vi "TEST_PumpController.vi"() -> ()   [LabVIEW 2024]
doc: "The purpose of this VI is for unit test of the Pump Controller"
uses:
  Control Definitions/Def PumpCtlRefs.ctl
  Control Definitions/Def PumpCtlOutputs.ctl
panel:
  in  "Pump Speed":enum16{"FAST", "SLOW", "CREEP", "STOP"}(ring)=enum."CREEP"
  in  "Bounds In":cluster{"Spec HI in":dbl, "Spec Lo in":dbl}={"Spec HI in"=7.5, "Spec Lo in"=7.4}
  out "outputs":T1={"PV"=2.1, "Done"=FALSE, "Over Fill"=FALSE, "Over Drain"=FALSE} {"PV" scale=0.0..10.0}
  in  "Level PV":dbl
  in  "Drain":bool
  in  "Fill":bool
  in  "Run Test":bool
  in  "Jog":bool
  in  "Pump CtlRef In":T2
  in  "Sim SwP":dbl=7.44 format="%_5g"
  in  "BinSearch":bool
  in  "Sim Pump":bool=TRUE
  in  "PV":dbl(slide)=2.1 scale=0.0..10.0
  in  "SP":dbl(slide)=7.448979591836735 scale=0.0..10.0
  in  "stop":bool
  # "PUMP CONTROLLER UNIT TEST\n1.  Perform these wiht Sim Pump ON\n2.  Turn on JOG;  Fill and Drain should fill and drain at the SLOW speed Rate\n3.  Over Fill ON when PV >=9 AND Over Drain ON when PV <= 1\n4.  With JOG OFF and BinSearch OFF and Run Test OFF, the PV should got to \n     the SP value +/- 0.001\n5,   With JOG OFF and BinSearch ON and Run Test OFF, the with Switch Point set \n     between Spec Hi in and Spec Lo in, the SwP Guess should settle on Switch \n     Point +/- 0.001 when the Done is ON."
  # "PUMP"
  # "From  Laser Sensor when not in Sim"
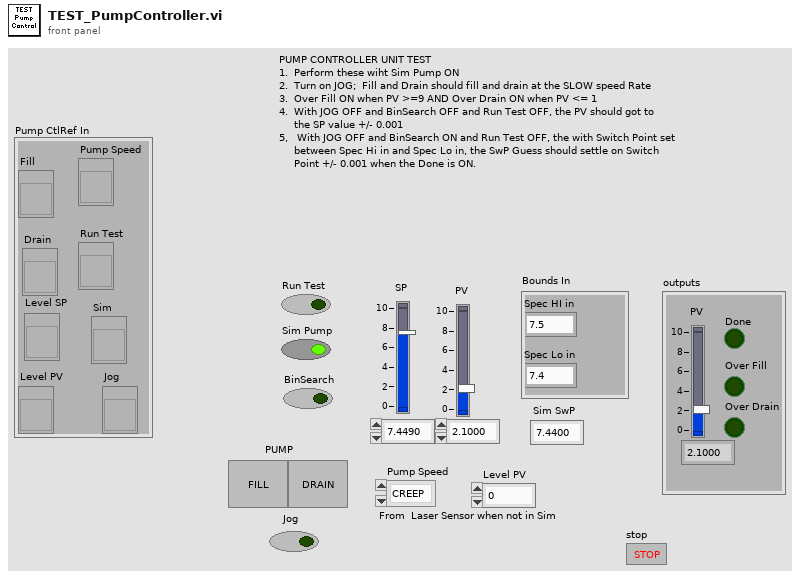
[diagram p1: front panel]
types:
  T1 = typedef "Def PumpCtlOutputs.ctl" = cluster{"PV":dbl, "Done":bool, "Over Fill":bool, "Over Drain":bool}
  T2 = typedef "Def PumpCtlRefs.ctl" = cluster{"Fill ":refnum<vi>, "Drain":refnum<vi>, "Level PV":refnum<vi>, "Pump Speed":refnum<vi>, "Run Test":refnum<vi>, "Sim":refnum<vi>, "Jog":refnum<vi>, "Level SP":refnum<vi>}
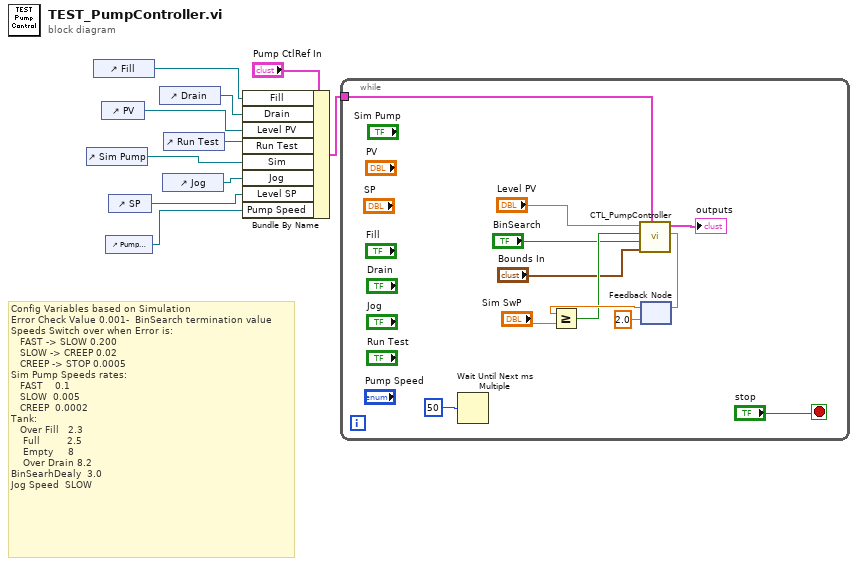
[diagram p0: block diagram]
diagram:
  # "Config Variables based on Simulation\nError Check Value 0.001-  BinSearch termination value\nSpeeds Switch over when Error is:\n   FAST -> SLOW 0.200\n   SLOW -> CREEP 0.02\n   CREEP -> STOP 0.0005\nSim Pump Speeds rates:\n   FAST    0.1\n   SLOW  0.005  \n   CREEP  0.0002\nTank:\n   Over Fill   2.3\n    Full         2.5\n    Empty     8\n    Over Drain 8.2\nBinSearhDealy  3.0\nJog Speed  SLOW"
  n1 = control-ref of="Sim Pump"() -> (w5:refnum<vi>)
  n2 = control-ref of="Fill"() -> (w2:refnum<vi>)
  n3 = control-ref of="PV"() -> (w4:refnum<vi>)
  n4 = control-ref of="Pump Speed"() -> (w1:refnum<vi>)
  n5 = control-ref of="SP"() -> (w8:refnum<vi>)
  n6 = control-ref of="Drain"() -> (w3:refnum<vi>)
  n7 = control-ref of="Jog"() -> (w6:refnum<vi>)
  n8 = control-ref of="Run Test"() -> (w7:refnum<vi>)
  n9 = Bundle By Name(cluster="Pump CtlRef In", "Fill"=w2, "Drain"=w3, "Level PV"=w4, "Run Test"=w7, "Sim"=w5, "Jog"=w6, "Level SP"=w8, "Pump Speed"=w1) -> (w9:T2)
  n10 = while {
    tunnel: w9 -> [w19]
    stop <- "stop" stop-if-true
    n11 = Wait Until Next ms Multiple(millisecond multiple=u32 50) -> ()  [unwired: 1 out]
    n12 = feedback #1(2.0 ("PV Out")) -> (w16:dbl)
    n13 = Greater Or Equal?(x=w16, y="Sim SwP") -> (x >= y?=w14:bool)
    n14 = call "CTL_PumpController.vi"("Pump CtlRef In"=w19, "Input cluster"="Bounds In", "BinSearch"="BinSearch", "Res Switched?"=w14, "Level PV"="Level PV") -> ("PV Out"=w17:dbl, "PumpCTLOutput"=→"outputs":T1)  [unwired: 5 in]
    n15 = feedback-in #1(w17) -> ()
  }
